vi "Loop_PCM_SEN.vi"() -> ()   [LabVIEW 2017, in "System_Status.lvlib"]
uses:
  System_Status.lvlib
  TypeDef/CLUSTER_PCM_Status.ctl
  _SHARE ALL/Global Share All/Global_STOP.vi
  Global_SEN Write_Data.vi
panel:
  out "Cycle Time (S)":dbl format="%.3g"
  in  "Target Time(ms)":u32=50
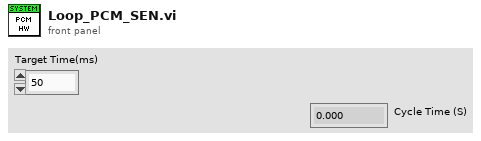
[diagram p1: front panel]
types:
  T1 = typedef "CLUSTER_PCM_Status.ctl" = cluster{"Current (A)":dbl, "All Solenoid Faults":bool[], "Input Voltage":dbl, "Solenoid Voltage":dbl, "Comp. Fault":bool}
  T2 = cluster{"PCM ID":i32, "Target Time(ms)":u32, "Current Time":timestamp, "Previous Time":timestamp, "Cycle Time (S)":dbl, "PCM Status":T1}
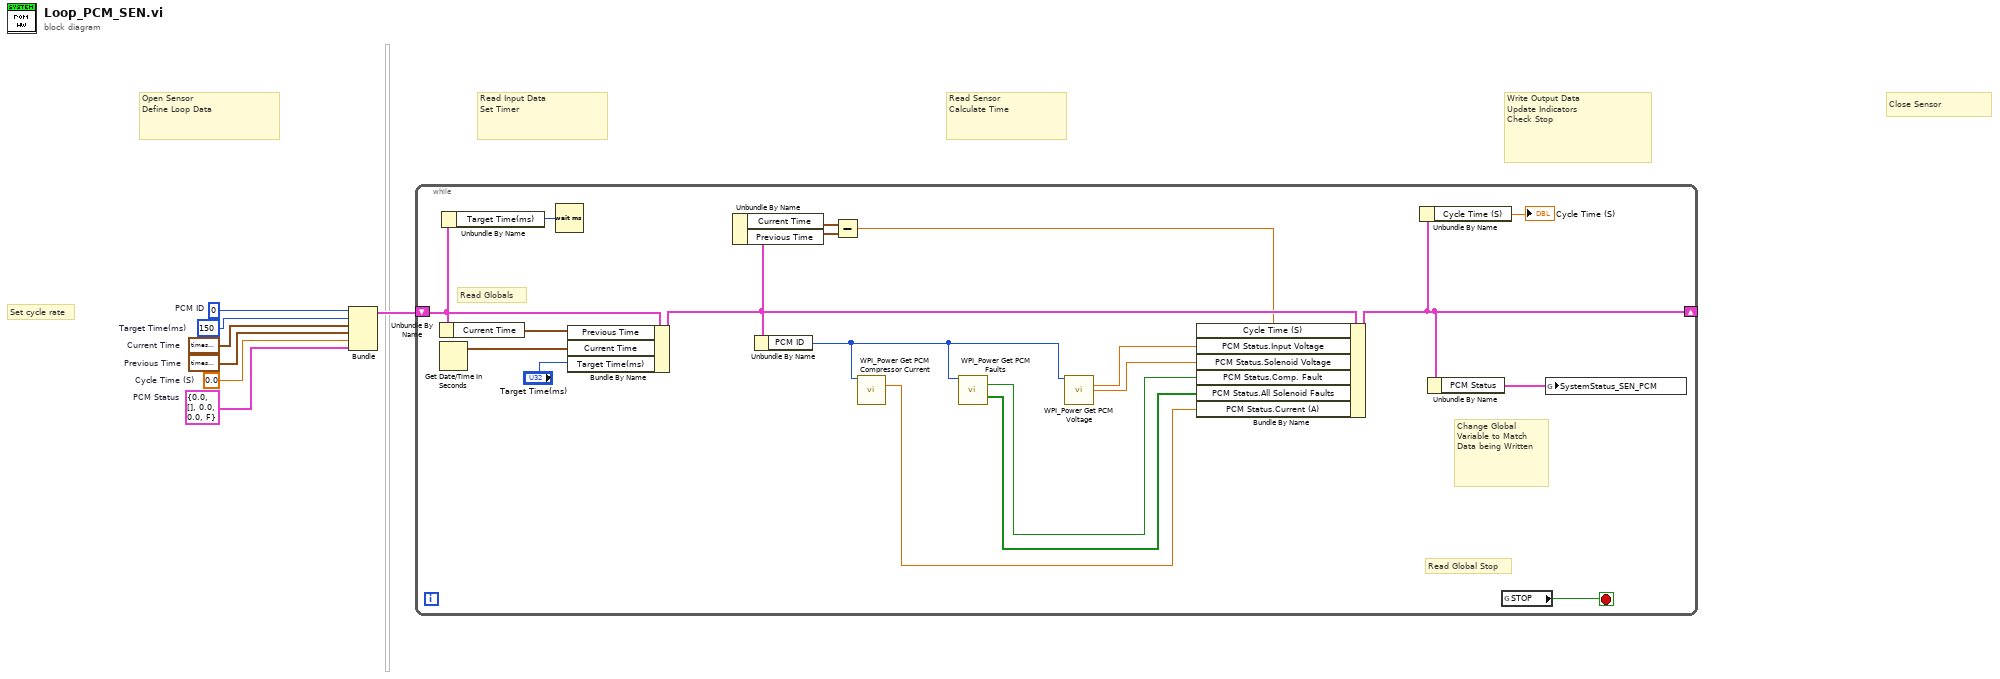
[diagram p0: block diagram]
diagram:
  w1 = T1 {"Current (A)"=0.0, "All Solenoid Faults"=[], "Input Voltage"=0.0, "Solenoid Voltage"=0.0, "Comp. Fault"=FALSE}  # PCM Status
  w2 = 0  # PCM ID
  w3 = 0.0  # Cycle Time (S)
  w7 = timestamp(0 s since 1904-01-01)  # Previous Time
  w6 = timestamp(0 s since 1904-01-01)  # Current Time
  w5 = u32 150  # Target Time(ms)
  # "Close Sensor"
  # "Write Output Data\nUpdate Indicators\nCheck Stop"
  # "Read Sensor\nCalculate Time"
  # "Read Input Data\nSet Timer"
  # "Open Sensor\nDefine Loop Data"
  # "Set cycle rate"
  n1 = Bundle("PCM ID"=w2, "Target Time(ms)"=w5, "Current Time"=w6, "Previous Time"=w7, "Cycle Time (S)"=w3, "PCM Status"=w1) -> (w4:T2)  [unwired: 1 in]
  n2 = while {
    shift-right: [w16] -> _
    shift-left: w4 -> [w18]
    stop <- w26 stop-if-true
    # "Change Global\nVariable to Match\nData being Written"
    # "Read Globals"
    # "Read Global Stop"
    n3 = Unbundle By Name(w18) -> ("Current Time"=w23:timestamp)
    n4 = Get Date/Time In Seconds() -> (seconds since 1Jan1904=w24:timestamp)
    n5 = Unbundle By Name(w18) -> ("Target Time(ms)"=w17:u32)
    n6 = Wait (ms)(milliseconds to wait=w17) -> ()  [unwired: 1 out]
    n7 = Bundle By Name(cluster=w18, "Previous Time"=w23, "Current Time"=w24, "Target Time(ms)"="Target Time(ms)") -> (w19:T2)
    n8 = Unbundle By Name(w19) -> ("Current Time"=w22:timestamp, "Previous Time"=w21:timestamp)
    n9 = Unbundle By Name(w19) -> ("PCM ID"=w13:i32)
    n10 = Subtract(x=w22, y=w21) -> (x-y=w14:dbl)
    n11 = call <vilib>:"WPI_Power Get PCM Compressor Current.vi"("Pneumatics Control Module (0)"=w13) -> ("current (A)"=w12:dbl)  [unwired: 13 in, 1 out]
    n12 = call <vilib>:"WPI_Power Get PCM Faults.vi"("Pneumatics Control Module (0)"=w13) -> ("Compressor Fault"=w9:bool, "All Solenoid Faults"=w11:bool[])  [unwired: 11 in, 2 out]
    n13 = call <vilib>:"WPI_Power Get PCM Voltage.vi"("Pneumatics Control Module (0)"=w13) -> ("Input Voltage"=w8:dbl, "Solenoid Voltage"=w10:dbl)  [unwired: 12 in, 1 out]
    n14 = Bundle By Name(cluster=w19, "Cycle Time (S)"=w14, "PCM Status.Input Voltage"=w8, "PCM Status.Solenoid Voltage"=w10, "PCM Status.Comp. Fault"=w9, "PCM Status.All Solenoid Faults"=w11, "PCM Status.Current (A)"=w12) -> (w16:T2)
    n15 = Unbundle By Name(w16) -> ("Cycle Time (S)"=→"Cycle Time (S)":dbl)
    n16 = Unbundle By Name(w16) -> ("PCM Status"=w25:T1)
    n17 = global read "Global_STOP.vi" "STOP"() -> (w26:bool)
    n18 = global write "Global_SEN Write_Data.vi" "SystemStatus_SEN_PCM"(w25) -> ()
  }
